vi "Write node type.vi"(8 "error in (no error)":errorcluster, 10 "node class":T1 items=["Unspecified"=0, "Object"=1, "Variable"=2, "Method"=4, "Object Type"=8, "Variable Type"=16, "Reference Type"=32, "Data Type"=64, "View"=128], 11 "UA Node in":refnum<class "UA Node.lvclass">) -> (0 "error out":errorcluster, 3 "UA Node out":refnum<class "UA Node.lvclass">)   [LabVIEW 2017, in "Browser Core.lvlib" / "UA Node.lvclass"]
uses:
  UA Node.lvclass
  Node Class.ctl
  UA Node.lvclass/UA Node.ctl
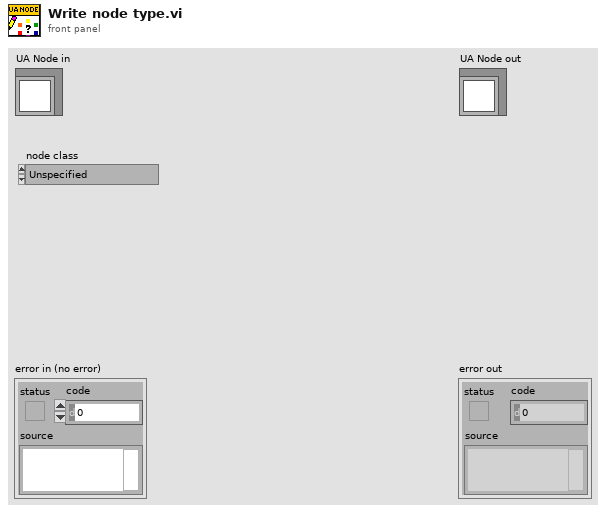
[diagram p1: front panel]
types:
  T1 = typedef "Browser Core.lvlib/UA Node.lvclass/Node Class.ctl" = u16
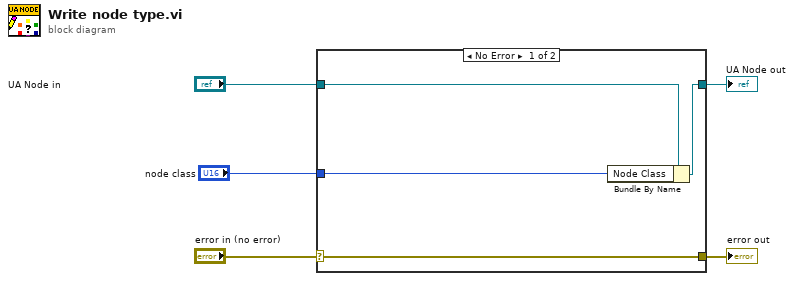
[diagram p0: block diagram]
diagram:
  n1 = case shown="No Error" "error in (no error)" {
    selector: "error in (no error)" -> [w9 w10]
    tunnel: [w9 w10] -> w4
    tunnel: [w7 w11] -> w2
    tunnel: "UA Node in" -> [w8 w11]
    tunnel: "node class" -> [w6 _]
    frame No Error {
      n2 = Bundle By Name(cluster=w8, "Node Class"=w6) -> (w7:refnum<class "UA Node.lvclass">)
    }
    frame Error {
    }
  }
  "error out" <- w4
  "UA Node out" <- w2
